vi "DSF.Engine.Debug Flags.FIFO.Set Infinite Timeouts.vi"(10 "infinite timeouts":bool, 11 "FIFO Debug Flags in":refnum<class "DSF.Engine.Debug Flags.FIFO.lvclass">) -> (3 "FIFO Debug Flags out":refnum<class "DSF.Engine.Debug Flags.FIFO.lvclass">)   [LabVIEW 2017, in "Data Sharing Framework Engine.lvlib" / "DSF.Engine.Debug Flags.FIFO.lvclass"]
uses:
  DSF.Engine.Debug Flags.FIFO.lvclass
  DSF.Engine.Debug Flags.FIFO.lvclass/DSF.Engine.Debug Flags.FIFO.ctl
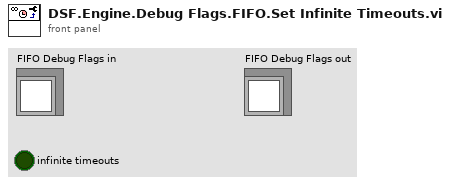
[diagram p1: front panel]
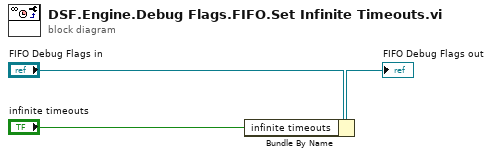
[diagram p0: block diagram]
diagram:
  n1 = Bundle By Name(cluster="FIFO Debug Flags in", "infinite timeouts"="infinite timeouts") -> (→"FIFO Debug Flags out":refnum<class "DSF.Engine.Debug Flags.FIFO.lvclass">)
